vi "_Load Markdown File.vi"(8 "Error In":errorcluster caption="error in (no error)", 11 "Path":path=path "D:/CSM Framework/Communicable-State-Machine/src/help/NEVSTOP/Communicable State Machine(CSM)") -> (0 "error out":errorcluster, 1 "Array 2":T1[](array[typedef]), 2 "Array":T2[](array[typedef]))   [LabVIEW 2017, in "csmdoc.lvlib"]
uses:
  csmdoc.lvlib
  _Typedef/DocElement.ctl
  _Typedef/DocNote.ctl
  _tool/_file/csm-file-support.lvlib
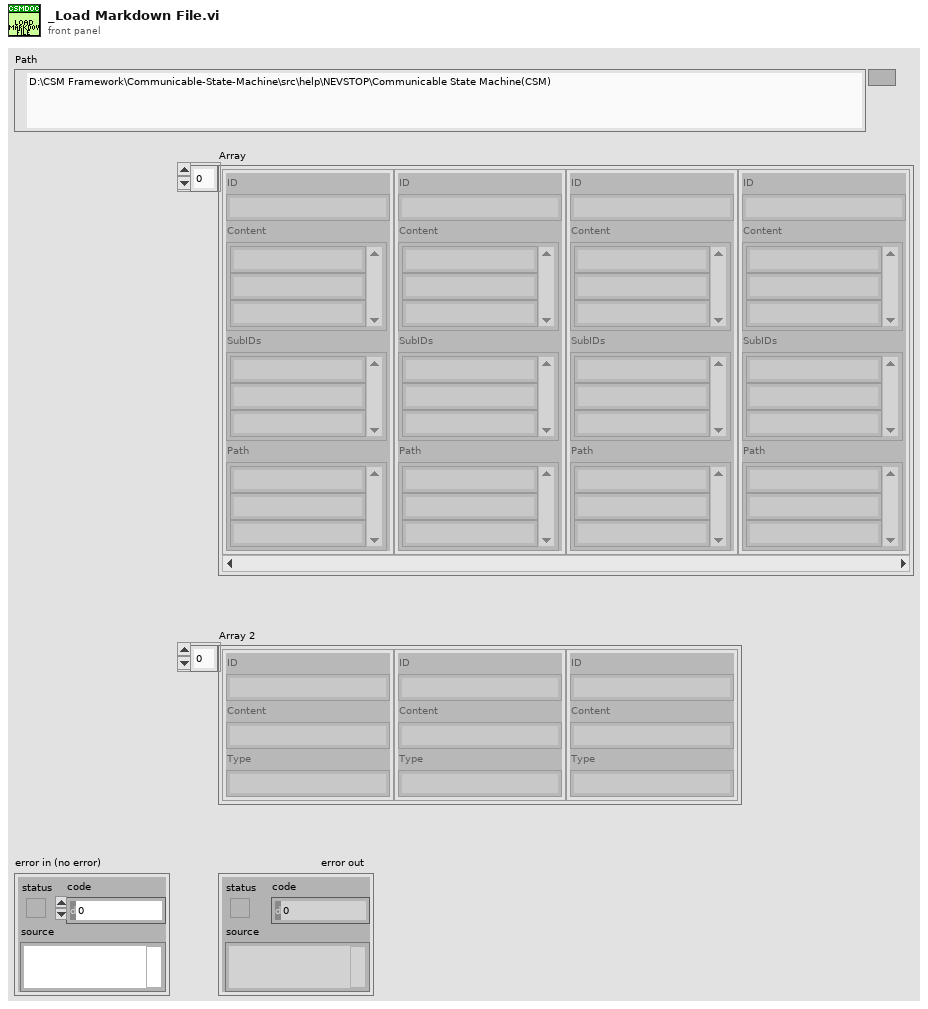
[diagram p1: front panel]
types:
  T1 = typedef "csmdoc.lvlib/DocNote.ctl" = cluster{"ID":string, "Content":string, "Type":string}
  T2 = typedef "csmdoc.lvlib/DocElement.ctl" = cluster{"ID":string, "Content":string[], "SubIDs":string[], "Path":string[]}
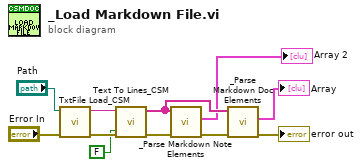
[diagram p0: block diagram]
diagram:
  n1 = call "TxtFile Load_CSM.vi"("error in (no error)"="Error In", "Path"="Path") -> ("error out"=w10:errorcluster, "Text"=w9:string)  [unwired: 8 in]
  n2 = call "Text To Lines_CSM.vi"("Remove Empty Lines? (T)"=FALSE ("Remove Empty Lines?(T)"), "error in (no error)"=w10, "String"=w9) -> ("error out"=w3:errorcluster, "Lines"=w6:string[])  [unwired: 7 in]
  n3 = call "_Parse Markdown Note Elements.vi"("Error in"=w3, "Lines"=w6) -> ("Error out"=w2:errorcluster, "Array"=→"Array 2":T1[])  [unwired: 7 in, 1 out]
  n4 = call "_Parse Markdown Doc Elements.vi"("Error in"=w2, "Lines"=w6) -> ("Error out"=→"error out":errorcluster, "Array"=→"Array":T2[])  [unwired: 7 in, 1 out]
